vi "oa_TV Extract Geometric Imperfection (Analog Tacho 1Chan).vi"(0 "analog tacho signal":waveform(dbl)={"t0"=timestamp(0 s since 1904-01-01), "dt"=0.0, "Y"=[]}, 1 "missing pulses? (no:F)":bool, 3 "reset? (F)":bool, 5 "threshold (auto)":dbl=inf format="%.2f", 7 "pulse/revolution":i32=1, 9 "hysteresis(0)":dbl format="%.2f", 11 "error in (no error)":errorcluster, 12 "pulse width (2)":i32=2, 14 "slope (Rising)":u16(ring) items=["Rising", "Falling"]) -> (4 "pulse positions":dbl[](array[numeric]), 8 "revulotion":i32, 10 "revulotion index":i32, 15 "error out":errorcluster)   [LabVIEW 2017, in "SoundVib_Torsional.lvlib"]
uses:
  <vilib>/addons/Sound and Vibration/Order Analysis/Torsional Vibration/SoundVib_Torsional.lvlib
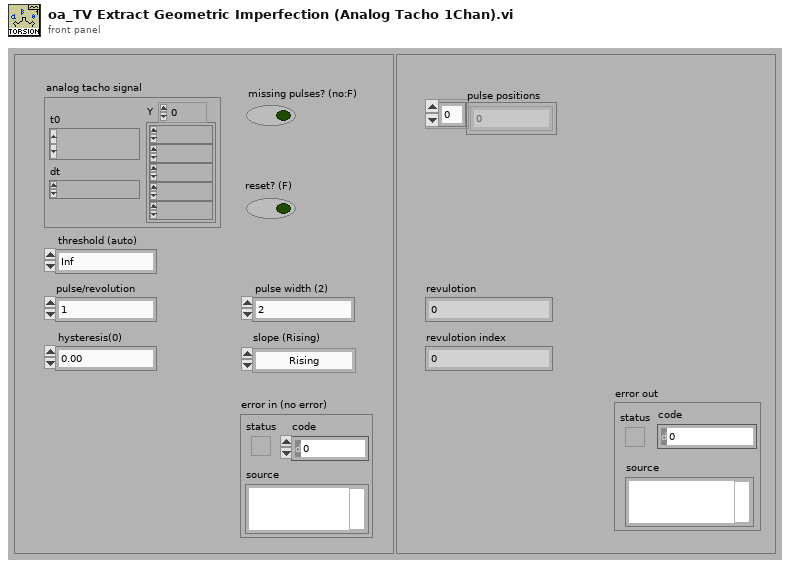
[diagram p1: front panel]
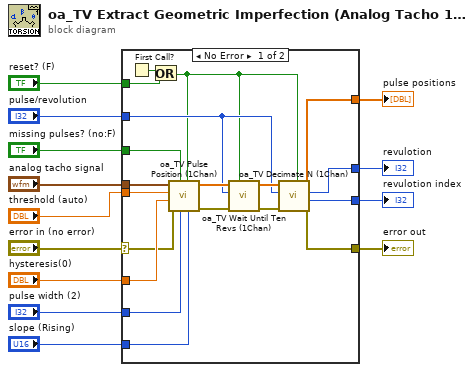
[diagram p0: block diagram]
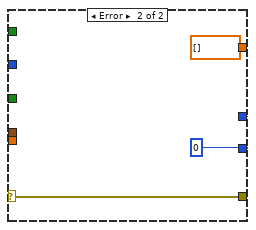
[diagram p2: hidden frame]
diagram:
  n1 = case shown="No Error" "error in (no error)" {
    selector: "error in (no error)" -> [w25 w35]
    tunnel: "analog tacho signal" -> [w32 _]
    tunnel: "pulse/revolution" -> [w19 _]
    tunnel: "threshold (auto)" -> [w31 _]
    tunnel: "pulse width (2)" -> [w30 _]
    tunnel: "slope (Rising)" -> [w29 _]
    tunnel: [w24 dbl[] [] ("Array")] -> w8
    tunnel: "hysteresis(0)" -> [w28 _]
    tunnel: [w27 w33] -> w6
    tunnel: [w16 w35] -> w4
    tunnel: "reset? (F)" -> [w17 _]
    tunnel: [w15 w33] -> w2
    tunnel: "missing pulses? (no:F)" -> [w14 _]
    frame No Error {
      n2 = First Call?() -> (First Call?: T/F=w26:bool)
      n3 = Or(x=w26, y=w17) -> (x .or. y?=w18:bool)
      n4 = call <vilib>:"oa_TV Pulse Position (1Chan).vi"("slope (Rising)"=w29, "reset? (F)"=w18, "pulse width (2)"=w30, "missing pulses? (no:F)"=w14, "error in (no error)"=w25, "hysteresis(0)"=w28, "threshold (auto)"=w31, "analog tacho signal"=w32) -> ("error out"=w23:errorcluster, "pulse positions [s]"=w22:dbl[])  [unwired: 1 in, 1 out]
      n5 = call <vilib>:"oa_TV Wait Until Ten Revs (1Chan).vi"("reset? (F)"=w18, "error in (no error)"=w23, "pulse/revolution"=w19, "pulse positions"=w22) -> ("error out"=w20:errorcluster, "pulse positions out"=w21:dbl[])  [unwired: 6 in]
      n6 = call <vilib>:"oa_TV Decimate N (1Chan).vi"("reset? (F)"=w18, "error in (no error)"=w20, "pulse/revolution"=w19, "pulse positions [s]"=w21) -> ("error out"=w16:errorcluster, "revolution index"=w27:i32, "revolution"=w15:i32, "pulse positions"=w24:dbl[])  [unwired: 4 in]
    }
    frame Error {
      w33 = 0 ("Revulotion")
    }
  }
  "revulotion" <- w2
  "pulse positions" <- w8
  "revulotion index" <- w6
  "error out" <- w4
